vi "Intervals Above Threshold.vi"(8 "Error In":errorcluster, 10 "Noise Threshold":dbl, 11 "Array in":dbl[](array[numeric])) -> (0 "Error Out":errorcluster, 3 "Intervals above Threshold":cluster{"start":i32, "end":i32}[](array[cluster]))   [LabVIEW 2021, in "Arrays.lvlib"]
uses:
  Arrays.lvlib
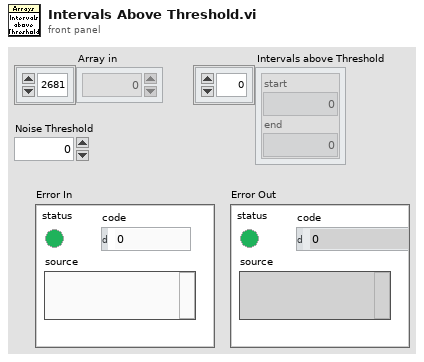
[diagram p1: front panel]
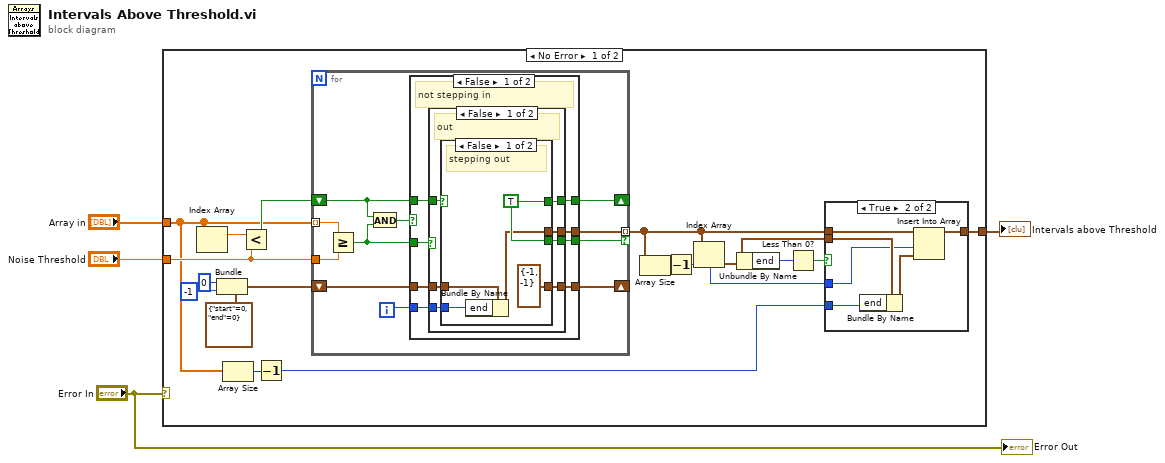
[diagram p0: block diagram]
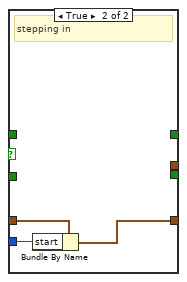
[diagram p5: hidden frame]
diagram:
  n1 = case shown="No Error" "Error In" {
    tunnel: [w21 _] -> w4
    tunnel: "Noise Threshold" -> [w11 _]
    tunnel: "Array in" -> [w7 _]
    frame No Error {
      n2 = Index Array(array=w7) -> (element=w10:dbl)  [unwired: 1 in]
      n3 = Bundle(cluster=cluster{"start":i32, "end":i32} {"start"=0, "end"=0}, "start"=0, "end"=-1) -> (w14:cluster{"start":i32, "end":i32})
      n4 = Array Size(array=w7) -> (size(s)=w6:i32)
      n5 = Less?(x=w10, y=w11) -> (x < y?=w9:bool)
      n6 = Decrement(x=w6) -> (x-1=w5:i32)
      n7 = for {
        tunnel: w7 -> [w39] mode=indexing
        tunnel: w11 -> [w38]
        shift-right: [w32] -> _
        shift-left: w9 -> [w33]
        shift-right: [w31] -> _
        shift-left: w14 -> [w36]
        tunnel: [w29] -> w19 mode=indexing if=w30
        i -> [w35]
        n8 = Greater Or Equal?(x=w39, y=w38) -> (x >= y?=w34:bool)
        n9 = And(x=w33, y=w34) -> (x .and. y?=w37:bool)
        n10 = case shown="False" w37 {
          tunnel: w36 -> [w44 w66]
          tunnel: w35 -> [w42 w65]
          tunnel: [w43 w64] -> w31
          tunnel: w34 -> [w47 _]
          tunnel: w33 -> [w46 _]
          tunnel: [w45 _] -> w32
          tunnel: [w41 _] -> w30
          tunnel: [w40 _] -> w29
          frame False {
            # "not stepping in"
            n11 = case shown="False" w47 {
              tunnel: w46 -> [w54 w63]
              tunnel: [w53 w63] -> w45
              tunnel: w44 -> [w52 w62]
              tunnel: [w51 w62] -> w43
              tunnel: w42 -> [w50 _]
              tunnel: [w49 _] -> w41
              tunnel: [w48 _] -> w40
              frame False {
                # "out"
                n12 = case shown="False" w54 {
                  selector: w54 -> [_ w61]
                  tunnel: [w57 w61] -> w53
                  tunnel: w52 -> [w59 w60]
                  tunnel: [cluster{"start":i32, "end":i32} {"start"=-1, "end"=-1} ("cluster") w60] -> w51
                  tunnel: w50 -> [w58 _]
                  tunnel: [w57 _] -> w49
                  tunnel: [w56 _] -> w48
                  frame False {
                    w57 = TRUE
                    # "stepping out"
                    n13 = Bundle By Name(cluster=w59, "end"=w58) -> (w56:cluster{"start":i32, "end":i32})
                  }
                  frame True {
                    # "still out"
                  }
                }
              }
              frame True {
                # "already in"
              }
            }
          }
          frame True {
            # "stepping in"
            n14 = Bundle By Name(cluster=w66, "start"=w65) -> (w64:cluster{"start":i32, "end":i32})
          }
        }
      }
      n15 = Array Size(array=w19) -> (size(s)=w16:i32)
      n16 = Decrement(x=w16) -> (x-1=w8:i32)
      n17 = Index Array(array=w19, index=w8) -> (element=w20:cluster{"start":i32, "end":i32})
      n18 = Unbundle By Name(w20) -> ("end"=w17:i32)
      n19 = Less Than 0?(x=w17) -> (x < 0?=w18:bool)
      n20 = case shown="True" w18 {
        tunnel: w19 -> [w22 w26]
        tunnel: [w22 w27] -> w21
        tunnel: w20 -> [_ w28]
        tunnel: w5 -> [_ w25]
        tunnel: w8 -> [_ w23]
        frame False {
        }
        frame True {
          n21 = Bundle By Name(cluster=w28, "end"=w25) -> (w24:cluster{"start":i32, "end":i32})
          n22 = Insert Into Array(array=w26, index=w23, new element=w24) -> (w27:cluster{"start":i32, "end":i32}[])
        }
      }
    }
    frame Error {
    }
  }
  "Intervals above Threshold" <- w4
  "Error Out" <- "Error In"
